vi "Set Scheme.vi"(10 "Scheme":string, 11 "URI in":refnum<class "URI.lvclass">) -> (3 "URI out":refnum<class "URI.lvclass">)   [LabVIEW 2020, in "URI.lvlib" / "URI.lvclass"]
uses:
  URI.lvclass
  URI.lvclass/URI.ctl
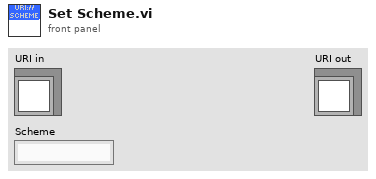
[diagram p1: front panel]
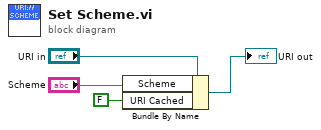
[diagram p0: block diagram]
diagram:
  n1 = Bundle By Name(cluster="URI in", "Scheme"="Scheme", "URI Cached"=FALSE ("String Cached")) -> (→"URI out":refnum<class "URI.lvclass">)
